vi "ConvolveFRF.vi"(9 "Sampling rate":u16=48000, 11 "Complex FRF":cluster{"t0":dbl, "dt":dbl, "Y":cdb[]}) -> (0 "Re":T1(graph), 1 "Im":T1(graph), 3 "Convolution":waveform(dbl)(graph))   [LabVIEW 2022 SP3]
uses:
  <vilib>/Analysis/2dsp.llb/Inverse Complex FFT.vi
  <vilib>/Analysis/2dsp.llb/1D Convolution (DBL).vi
  <vilib>/measure/maresamp.llb/Resample Waveform (single shot).vi
  <vilib>/Analysis/NI_AALPro.lvlib
  <vilib>/Analysis/NI_AALBase.lvlib
  <vilib>/measure/NI_MAPro.lvlib
panel:
  in  "Full?":bool
  out "Waveform Graph 4":dbl[](graph)
  out "FRF":cluster{"t0":dbl, "dt":dbl, "Y":dbl[]}(graph)
  in  "musical piece":waveform(dbl)[](graph)=[{"t0"=timestamp(0 s since 1904-01-01), "dt"=2.0833333333333333e-05, "Y"=array[288010 elements]}, {"t0"=timestamp(0 s since 1904-01-01), "dt"=2.0833333333333333e-05, "Y"=array[288010 elements]}]
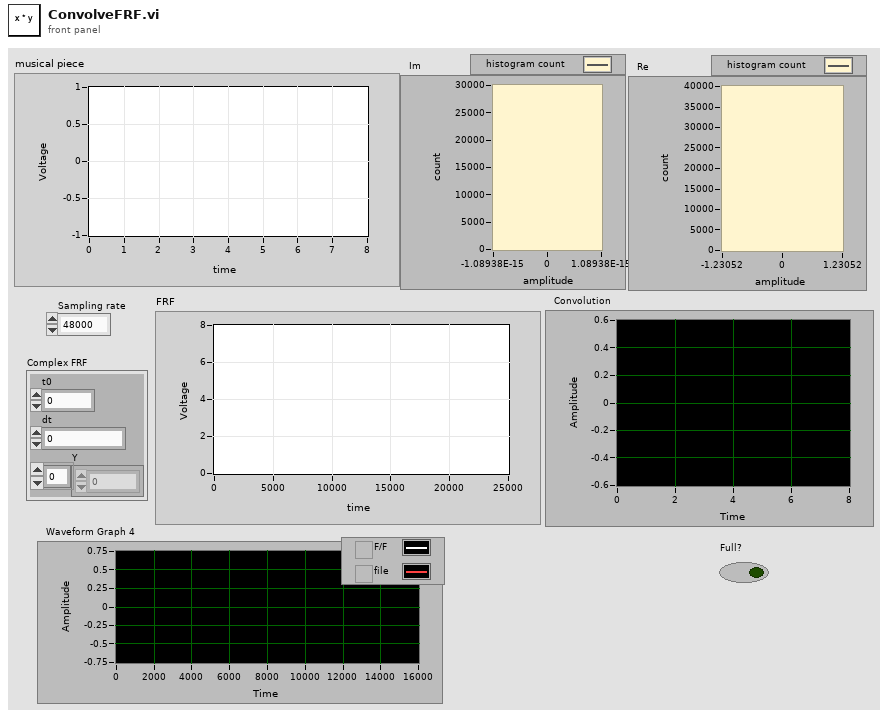
[diagram p1: front panel]
types:
  T1 = cluster{"X Values":dbl[], "Histogram: h(x)":i32[]}
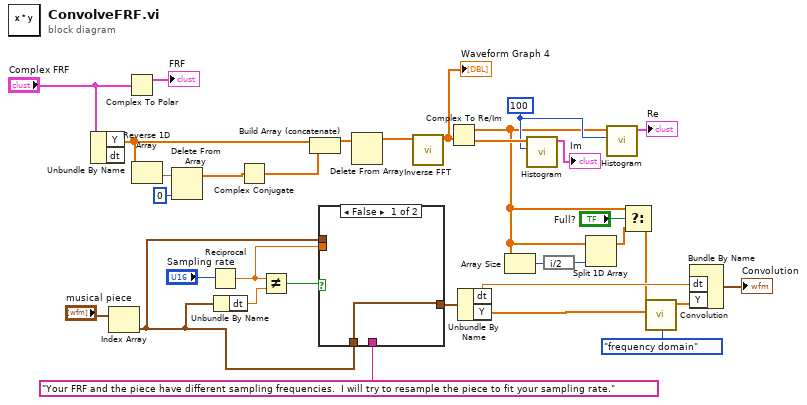
[diagram p0: block diagram]
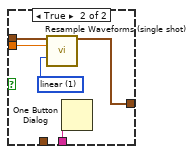
[diagram p2: hidden frame]
diagram:
  w26 = 100 ("intervals")
  n1 = Unbundle By Name("Complex FRF") -> ("Y"=w10:cdb[])  [unwired: 1 out]
  n2 = Index Array(array="musical piece") -> (element=w20:waveform(dbl))  [unwired: 1 in]
  n3 = Complex To Polar(r * e^(i*theta)="Complex FRF") -> (r=→"FRF":cluster{"t0":dbl, "dt":dbl, "Y":dbl[]})  [unwired: 1 out]
  n4 = Reverse 1D Array(array=w10) -> (reversed array=w31:cdb[])
  n5 = Delete From Array(array=w31, index=0) -> (array with subset deleted=w2:cdb[])  [unwired: 1 in, 1 out]
  n6 = Reciprocal(x="Sampling rate") -> (1/x=w13:dbl)
  n7 = Unbundle By Name(w20) -> ("dt"=w14:dbl)
  n8 = Complex Conjugate(1:w2) -> (0:w1:cdb[])
  n9 = Not Equal?(x=w13, y=w14) -> (x != y?=w23:bool)
  n10 = Build Array (concatenate)(w10, w1) -> (w12:cdb[])
  n11 = case shown="False" w23 {
    tunnel: "Your FRF and the piece have different sampling frequencies.  I will try to resample the piece to fit your sampling rate." ("message") -> [_ w39]
    tunnel: w20 -> [_ w38]
    tunnel: [w34 w36] -> w17
    tunnel: w20 -> [w34 _]
    tunnel: w13 -> [_ w35]
    frame False {
    }
    frame True {
      w37 = u16 1 items=["coerce", "linear", "spline", "FIR filter"] ("interpolation mode")
      n12 = call-poly <vilib>:"Resample Waveforms (single shot).vi"("waveform in"=w38, "dt"=w35, "interpolation mode"=w37) -> ("resampled waveform out"=w36:waveform(dbl))  [unwired: 9 in, 3 out]
      n13 = One Button Dialog(message=w39) -> ()  [unwired: 1 in, 1 out]
    }
  }
  n14 = Delete From Array(array=w12) -> (array with subset deleted=w30:cdb[])  [unwired: 2 in, 1 out]
  n15 = call-poly <vilib>:"Inverse FFT.vi"("FFT {X}"=w30) -> ("X"=w11:cdb[])  [unwired: 9 in, 1 out]
  "Waveform Graph 4" <- w11
  n16 = Complex To Re/Im(x + iy=w11) -> (x=w6:dbl[], y=w27:dbl[])
  n17 = Unbundle By Name(w17) -> ("dt"=w15:dbl, "Y"=w21:dbl[])
  n18 = Array Size(array=w6) -> (size(s)=w9:i32)
  n19 = call <vilib>:"Histogram.vi"("intervals"=w26, "X"=w27) -> ("Histogram Graph"=→"Im":T1)  [unwired: 6 in, 3 out]
  n20 = expression code="i/2"(w9) -> (w8:i32)
  n21 = Split 1D Array(array=w6, index=w8) -> (first subarray=w5:dbl[])  [unwired: 1 out]
  n22 = call <vilib>:"Histogram.vi"("intervals"=w26, "X"=w6) -> ("Histogram Graph"=→"Re":T1)  [unwired: 6 in, 3 out]
  n23 = Select(t=w6, s="Full?", f=w5) -> (s? t:f=w4:dbl[])
  n24 = call-poly <vilib>:"Convolution.vi"("algorithm"=enum32{"direct", "frequency domain"}."frequency domain", "Y"=w21, "X"=w4) -> ("X * Y"=w28:dbl[])  [unwired: 7 in, 1 out]
  n25 = Bundle By Name("dt"=w15, "Y"=w28) -> (→"Convolution":waveform(dbl))  [unwired: 1 in]
